vi "Test Buffer to Elec Grid.vi"() -> ()   [LabVIEW 2017]
panel:
  out "Array 2":bool[][](array[boolean])
  in  "Array":bool[][](array[boolean])
  in  "Bitmask":u64 format="%064b"
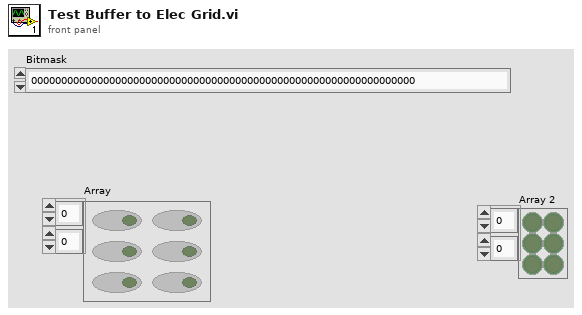
[diagram p1: front panel]
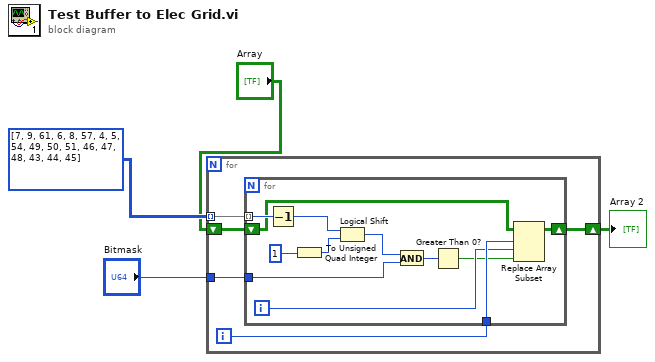
[diagram p0: block diagram]
diagram:
  n1 = for {
    tunnel: u8[][] [[7, 9, 61], [6, 8, 57], [4, 5, 54], [49, 50, 51], [46, 47, 48], [43, 44, 45]] -> [w9] mode=indexing
    tunnel: "Bitmask" -> [w8]
    shift-right: [w5] -> w1
    shift-left: "Array" -> [w6]
    i -> [w7]
    n2 = for {
      tunnel: w9 -> [w21] mode=indexing
      tunnel: w8 -> [w19]
      tunnel: w7 -> [w14]
      shift-right: [w10] -> w5
      shift-left: w6 -> [w13]
      i -> [w12]
      n3 = Decrement(x=w21) -> (x-1=w20:u8)
      n4 = To Unsigned Quad Integer(1:u32 1 ("x")) -> (0:w16:u64)
      n5 = Logical Shift(y=w20, x=w16) -> (x << y=w18:u64)
      n6 = And(x=w18, y=w19) -> (x .and. y?=w15:u64)
      n7 = Greater Than 0?(x=w15) -> (x > 0?=w11:bool)
      n8 = Replace Array Subset(array=w13, new element=w11, index (row)=w14, index (col)=w12) -> (w10:bool[][])
    }
  }
  "Array 2" <- w1
